vi "obtain sensor data.vi"(11 "Template in":refnum<class "Template.lvclass">) -> (0 "error out":errorcluster, 3 "Template out":refnum<class "Template.lvclass">)   [LabVIEW 2020, in "Template.lvlib" / "Template.lvclass"]
doc: "Reads the information from the sensor and stores it in the parent class' private data"
uses:
  Template.lvclass
  Template.lvclass/Template.ctl
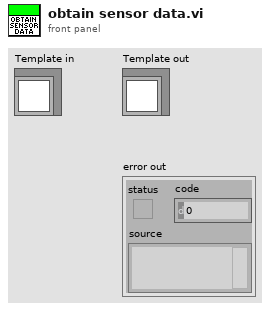
[diagram p1: front panel]
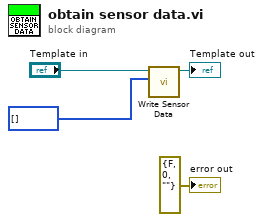
[diagram p0: block diagram]
diagram:
  n1 = call "Write Sensor Data.vi"("Sensor Data"=u8[] [], "Template in"="Template in") -> ("Template out"=→"Template out":refnum<class "Template.lvclass">)  [unwired: 9 in]
  "error out" <- errorcluster {"status"=FALSE, "code"=0, "source"=""} ("error out")
